vi "re_LuaVIEW Task State Machine.vi"   [LabVIEW 2012]
doc: "Implements a LuaVIEW task execution management: script compilation, execution, and default signal handling."
uses:
  typedefs/t_LuaVIEW Task States.ctl
  typedefs/t_LuaVIEW Task State Methods.ctl
  typedefs/t_LuaVIEW Task Signals.ctl
  typedefs/et_LuaVIEW CIN Actions.ctl
  typedefs/t_LuaVIEW Task Modes.ctl
  typedefs/t_LuaVIEW Task State Instantiator Methods.ctl
  typedefs/t_LuaVIEW Task List Methods.ctl
types:
  T1 = typedef "t_LuaVIEW Task States.ctl" = enum16{"handle signals", "test confirm", "test stop", "test swap", "test pause", "test resume", "sleep", "execute", "initialize", "list self", "set refs", "error", "stop"}
  T2 = typedef "t_LuaVIEW Task Signals.ctl" = enum32{"resume", "pause", "swap", "stop", "confirm"}
  T3 = typedef "t_LuaVIEW Task State Methods.ctl" = enum16{"cleanup", "set initial", "set mode", "set active mode", "set error", "get task info", "get script info", "set signal", "clear signal", "test handled", "test delegated", "test signal", "handle signal", "delegate signal", "allow signal", "disallow signal", "disallow all", "signals?", "delegated signals?", "protection++", "protection--", "protection=0", "message", "next message", "pop message", "message available?", "force stop", "set swap preps", "apply swap preps"}
  T4 = typedef "et_LuaVIEW CIN Actions.ctl" = enum16{"checksynopsis", "_open", "_registerpublic", "_registerexport", "__never_an_error_result_ns", "luaversion", "cinversion", "_totals", "_taskcount", "pathological", "_unregnextpublic", "registryusecount", "__per_state_actions", "regsetprivate", "regsetindex", "regsetmodule", "_revokeexports", "_usepublic", "prepare", "compile", "execute", "call", "unregstaterefs", "_close", "pullboolean", "pullnumber", "pullI8", "pullU8", "pullI16", "pullU16", "pullI32", "pullU32", "pullobject", "pullrefnum", "pullstring", "pullflat", "pushflat", "pushobject", "getattribute", "setattribute", "stacktostring", "_startyieldtest", "_endyieldtest", "_pollprintbuffer", "__never_an_error_result_ps", "_pollexport", "setclone", "forcecleanup", "gettop", "clearstack", "insert", "pushboolean", "pushnumber", "pushrefnum", "pushstring", "pushnil", "pushvalue", "gettaskref", "settaskref"}
  T5 = typedef "t_LuaVIEW Task Modes.ctl" = enum16{"initializing", "running", "executing", "paused", "error", "swapping"}
  T6 = typedef "t_LuaVIEW Task State Instantiator Methods.ctl" = enum16{"instantiate", "isset", "retrieve"}
  T7 = typedef "t_LuaVIEW Task List Methods.ctl" = enum16{"clear list", "add", "test", "remove", "get ref", "get task info", "get list", "get script info", "ongoing?", "resume", "pause", "stop", "confirm", "message"}
  T8 = typedef "t_LuaVIEW Task State Pane.ctl" = refnum<vi>
  T9 = typedef "t_LuaVIEW Reference.ctl" = refnum<k1>
  T10 = typedef "LuaVIEW Task Info.ctl" = cluster{"main script":string, "identifier":string, "class":string, "description":string, "mode":T5, "handler":string, "LuaVIEW reference":T9, "scripts":i32, "hide":bool, "active":bool, "error msg":string, "defer":bool, "launch":enum16{"asynchronous", "manual", "synchronous"}, "main path valid":bool, "start time":dbl, "swap time":dbl, "task VI":refnum<vi>, "prefsys":enum32{"invalid execution system", "user interface", "standard", "instrument i/o", "data acquisition", "other 1", "other 2", "same as caller"}, "priority":enum32{"invalid priority", "background priority", "normal priority", "above normal priority", "high priority", "time critical priority", "subroutine"}, "signal flags":u32, "allow mask":u32, "handle mask":u32, "disallow manual":bool}
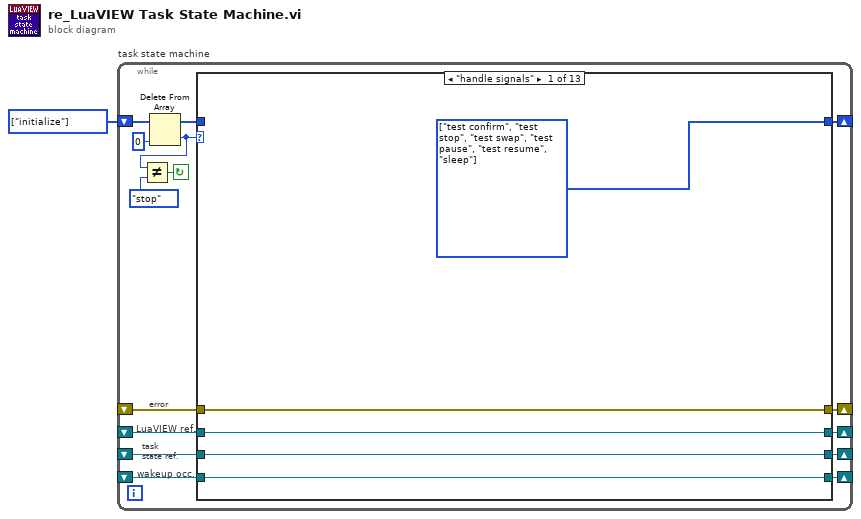
[diagram p0: block diagram]
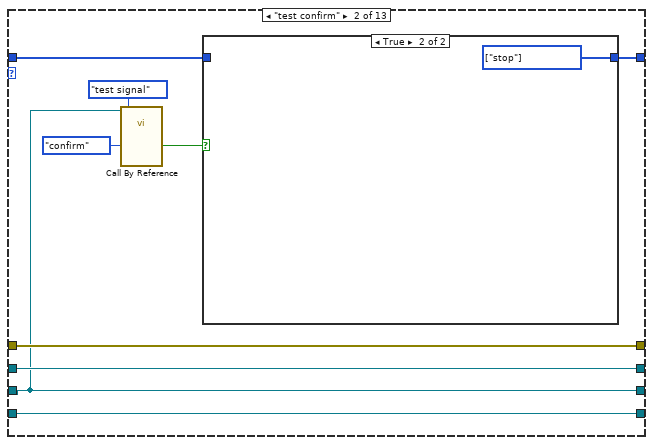
[diagram p2: hidden frame]
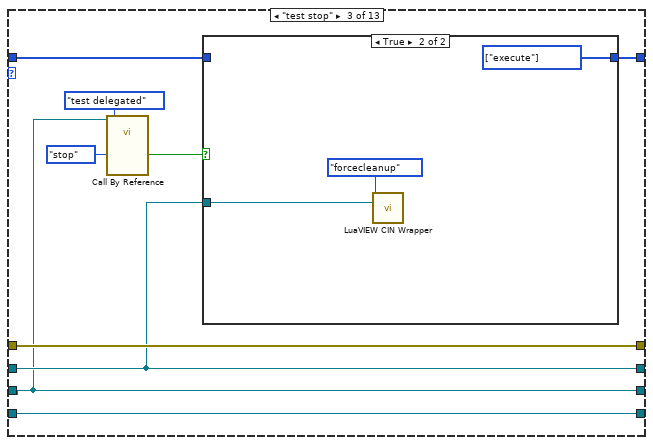
[diagram p4: hidden frame]
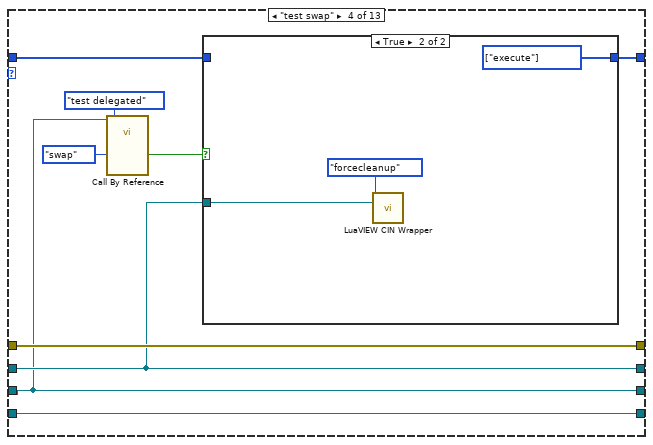
[diagram p6: hidden frame]
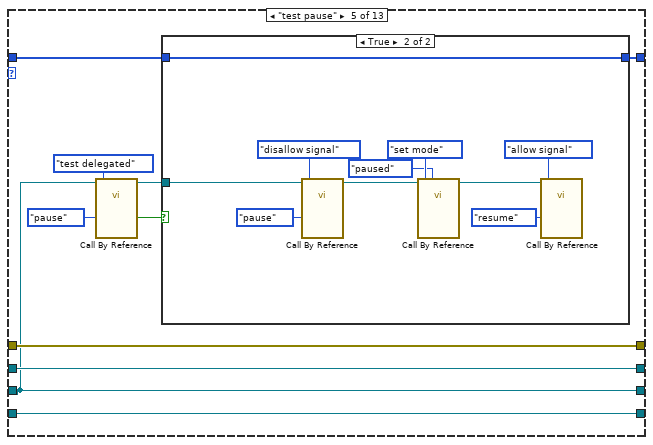
[diagram p8: hidden frame]
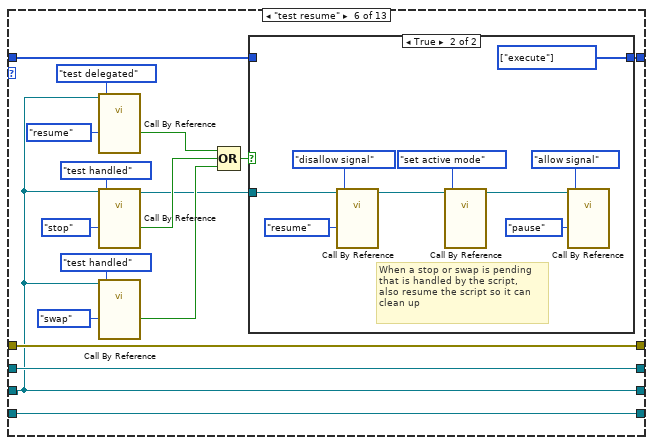
[diagram p10: hidden frame]
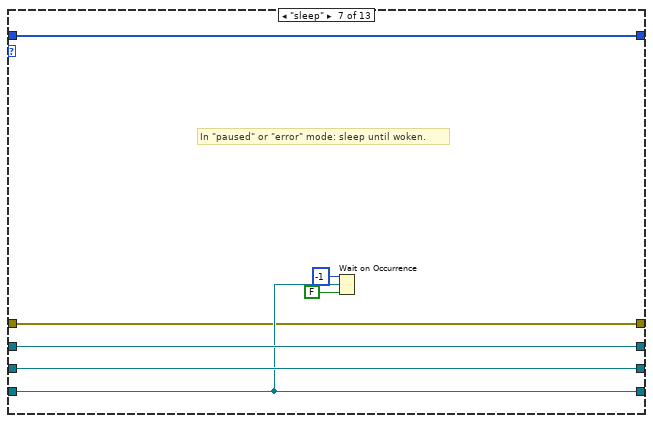
[diagram p12: hidden frame]
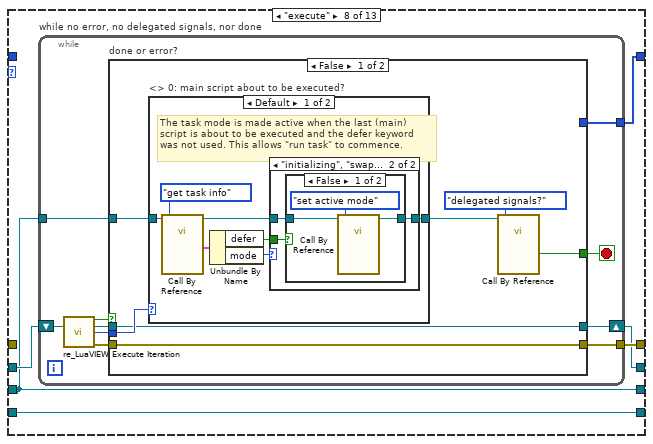
[diagram p13: hidden frame]
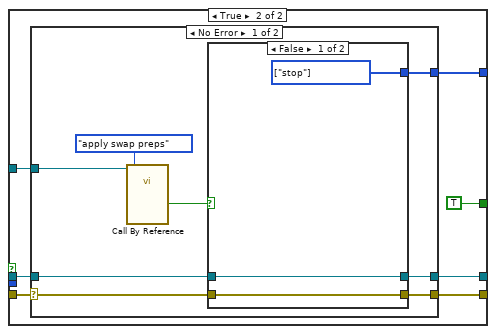
[diagram p17: hidden frame]
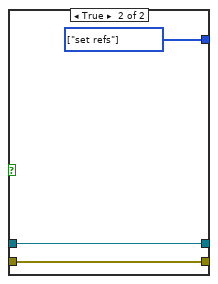
[diagram p18: hidden frame]
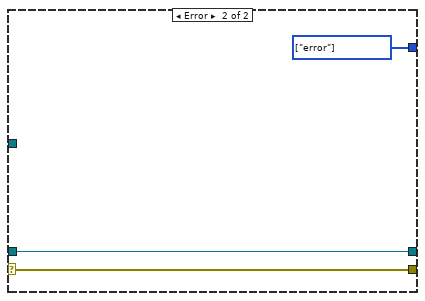
[diagram p19: hidden frame]
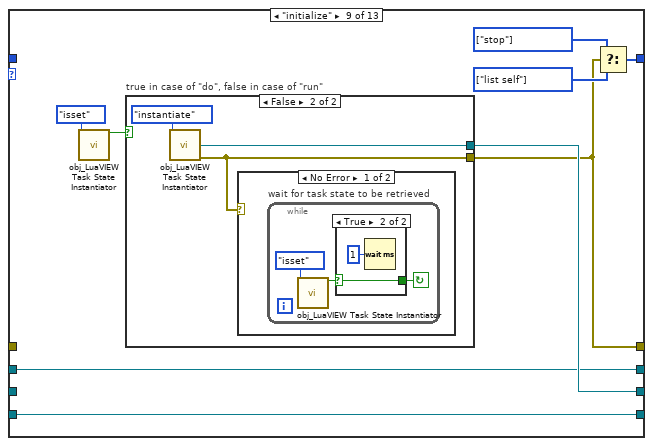
[diagram p20: hidden frame]
diagram:
  w1 = T1[] [enum."initialize"] items=["handle signals", "test confirm", "test stop", "test swap", "test pause", "test resume", "sleep", "execute", "initialize", "list self", "set refs", "error", "stop"] ("Array Constant")
  n1 = while "task state machine" {
    shift-left: w1 -> [w14]
    shift-right: [w7] -> _
    shift-right: [w11] -> _
    shift-left: _ -> [w8]
    shift-right: [w3] -> _
    shift-left: _ -> [w4]
    shift-right: [w10] -> _
    shift-left: _ -> [w9]
    shift-right: [w6] -> _
    shift-left: _ -> [w5]
    stop <- w16 continue-if-true
    # "error"
    # "LuaVIEW ref."
    # "task\nstate ref."
    # "wakeup occ."
    n2 = Delete From Array(array=w14, index=0) -> (deleted portion=w2:T1, array with subset deleted=w13:T1[])  [unwired: 1 in]
    n3 = Not Equal?(x=w2, y=t_LuaVIEW_Task_States."stop" ("states")) -> (x != y?=w16:bool)
    n4 = case "Case" shown="\"handle signals\"" w2 {
      tunnel: [w17 w27 w39 w52 w65 w93 w107 w115 w183 w199 w211 w218 w228] -> w7
      tunnel: w13 -> [_ w28 w40 w53 w66 w94 w107 _ _ _ _ _ w228]
      tunnel: [w20 w25 w36 w49 w60 w81 w112 w114 w180 w202 w208 w214 w222] -> w11
      tunnel: [w19 w29 w41 w54 w67 w95 w109 w117 w177 w198 w213 w220 w227] -> w10
      tunnel: w9 -> [w19 w29 w41 w54 w67 w95 w109 w117 w177 _ w213 w220 w227]
      tunnel: w8 -> [w20 w25 w36 w49 w60 w81 w112 w114 _ w202 w208 w214 w223]
      tunnel: [w21 w30 w37 w50 w68 w96 w113 w118 w178 w201 w206 w221 w226] -> w3
      tunnel: w4 -> [w21 w30 w37 w50 w68 w96 w113 w116 w178 w201 _ w221 w226]
      tunnel: [w18 w26 w38 w51 w64 w92 w108 w119 w179 w200 w212 w219 w225] -> w6
      tunnel: w5 -> [w18 w26 w38 w51 w64 w92 w108 _ _ w200 w212 w219 w225]
      frame "handle signals" {
        w17 = T1[] [enum."test confirm", enum."test stop", enum."test swap", enum."test pause", enum."test resume", enum."sleep"] items=["handle signals", "test confirm", "test stop", "test swap", "test pause", "test resume", "sleep", "execute", "initialize", "list self", "set refs", "error", "stop"] ("Array Constant")
      }
      frame "test confirm" {
        n5 = call-by-ref "?"(reference=w25, "method"=t_LuaVIEW_Task_State_Methods."test signal", "signal"=t_LuaVIEW_Task_Signals."confirm") -> ("set/available/pending"=w22:bool)  [unwired: 10 in, 6 out]
        n6 = case shown="True" w22 {
          tunnel: w28 -> [w31 _]
          tunnel: [w31 w32] -> w27
          frame False {
          }
          frame True {
            w32 = T1[] [enum."stop"] items=["handle signals", "test confirm", "test stop", "test swap", "test pause", "test resume", "sleep", "execute", "initialize", "list self", "set refs", "error", "stop"] ("Array Constant")
          }
        }
      }
      frame "test stop" {
        n7 = call-by-ref "?"(reference=w36, "method"=t_LuaVIEW_Task_State_Methods."test delegated", "signal"=t_LuaVIEW_Task_Signals."stop") -> ("set/available/pending"=w35:bool)  [unwired: 10 in, 6 out]
        n8 = case shown="True" w35 {
          tunnel: w40 -> [w42 _]
          tunnel: [w42 w45] -> w39
          tunnel: w37 -> [_ w43]
          frame False {
          }
          frame True {
            w45 = T1[] [enum."execute"] items=["handle signals", "test confirm", "test stop", "test swap", "test pause", "test resume", "sleep", "execute", "initialize", "list self", "set refs", "error", "stop"] ("Array Constant")
            n9 = call "LuaVIEW CIN Wrapper.vi"("action"=et_LuaVIEW_CIN_Actions."forcecleanup", "LuaVIEW reference in"=w43) -> ()  [unwired: 13 in, 1 out]
          }
        }
      }
      frame "test swap" {
        n10 = call-by-ref "?"(reference=w49, "method"=t_LuaVIEW_Task_State_Methods."test delegated", "signal"=t_LuaVIEW_Task_Signals."swap") -> ("set/available/pending"=w48:bool)  [unwired: 10 in, 6 out]
        n11 = case shown="True" w48 {
          tunnel: w53 -> [w55 _]
          tunnel: [w55 w58] -> w52
          tunnel: w50 -> [_ w56]
          frame False {
          }
          frame True {
            w58 = T1[] [enum."execute"] items=["handle signals", "test confirm", "test stop", "test swap", "test pause", "test resume", "sleep", "execute", "initialize", "list self", "set refs", "error", "stop"] ("Array Constant")
            n12 = call "LuaVIEW CIN Wrapper.vi"("action"=et_LuaVIEW_CIN_Actions."forcecleanup", "LuaVIEW reference in"=w56) -> ()  [unwired: 13 in, 1 out]
          }
        }
      }
      frame "test pause" {
        n13 = call-by-ref "?"(reference=w60, "method"=t_LuaVIEW_Task_State_Methods."test delegated", "signal"=t_LuaVIEW_Task_Signals."pause") -> (reference out=w59:T8, "set/available/pending"=w61:bool)  [unwired: 10 in, 5 out]
        n14 = case shown="True" w61 {
          tunnel: w66 -> [w69 w79]
          tunnel: [w69 w79] -> w65
          tunnel: w59 -> [_ w72]
          frame False {
          }
          frame True {
            n15 = call-by-ref "?"(reference=w72, "method"=t_LuaVIEW_Task_State_Methods."disallow signal", "signal"=t_LuaVIEW_Task_Signals."pause") -> (reference out=w71:T8)  [unwired: 10 in, 6 out]
            n16 = call-by-ref "?"(reference=w71, "method"=t_LuaVIEW_Task_State_Methods."set mode", "mode {set mode}"=t_LuaVIEW_Task_Modes."paused" ("mode")) -> (reference out=w70:T8)  [unwired: 10 in, 6 out]
            n17 = call-by-ref "?"(reference=w70, "method"=t_LuaVIEW_Task_State_Methods."allow signal", "signal"=t_LuaVIEW_Task_Signals."resume") -> ()  [unwired: 10 in, 7 out]
          }
        }
      }
      frame "test resume" {
        n18 = call-by-ref "?"(reference=w81, "method"=t_LuaVIEW_Task_State_Methods."test delegated", "signal"=t_LuaVIEW_Task_Signals."resume") -> ("set/available/pending"=w82:bool)  [unwired: 10 in, 6 out]
        n19 = call-by-ref "?"(reference=w81, "method"=t_LuaVIEW_Task_State_Methods."test handled", "signal"=t_LuaVIEW_Task_Signals."stop") -> (reference out=w80:T8, "set/available/pending"=w85:bool)  [unwired: 10 in, 5 out]
        n20 = call-by-ref "?"(reference=w81, "method"=t_LuaVIEW_Task_State_Methods."test handled", "signal"=t_LuaVIEW_Task_Signals."swap") -> ("set/available/pending"=w88:bool)  [unwired: 10 in, 6 out]
        n21 = Compound Arithmetic op=OR(w82, w85, w88) -> (w91:bool)
        n22 = case shown="True" w91 {
          tunnel: w94 -> [w97 _]
          tunnel: [w97 w106] -> w93
          tunnel: w80 -> [_ w98]
          frame False {
          }
          frame True {
            w106 = T1[] [enum."execute"] items=["handle signals", "test confirm", "test stop", "test swap", "test pause", "test resume", "sleep", "execute", "initialize", "list self", "set refs", "error", "stop"] ("Array Constant")
            # "When a stop or swap is pending\nthat is handled by the script,\nalso resume the script so it can\nclean up"
            n23 = call-by-ref "?"(reference=w98, "method"=t_LuaVIEW_Task_State_Methods."disallow signal", "signal"=t_LuaVIEW_Task_Signals."resume") -> (reference out=w100:T8)  [unwired: 10 in, 6 out]
            n24 = call-by-ref "?"(reference=w100, "method"=t_LuaVIEW_Task_State_Methods."set active mode") -> (reference out=w99:T8)  [unwired: 11 in, 6 out]
            n25 = call-by-ref "?"(reference=w99, "method"=t_LuaVIEW_Task_State_Methods."allow signal", "signal"=t_LuaVIEW_Task_Signals."pause") -> ()  [unwired: 10 in, 7 out]
          }
        }
      }
      frame "sleep" {
        # "In \"paused\" or \"error\" mode: sleep until woken."
        n26 = Wait on Occurrence(1:FALSE ("ignore previous (T)"), 2:w109, 3:-1 ("ms timeout (-1)")) -> ()  [unwired: 1 out]
      }
      frame "execute" {
        n27 = while "while no error, no delegated signals, nor done" {
          shift-right: [w129] -> w118
          shift-left: w116 -> [w123]
          tunnel: [w128] -> w119
          tunnel: [w121] -> w115
          tunnel: w114 -> [w120]
          stop <- w127 stop-if-true
          n28 = call "re_LuaVIEW Execute Iteration.vi"("LuaVIEW reference in"=w123) -> ("last?"=w122:bool, "LuaVIEW reference out"=w125:T9, "function index"=w126:i32, "final error"=w124:errorcluster)  [unwired: 11 in]
          n29 = case "done or error?" shown="False" w122 {
            tunnel: [w135 w155] -> w129
            tunnel: [w134 w158] -> w128
            tunnel: [w133 TRUE] -> w127
            tunnel: w126 -> [w136 _]
            tunnel: w125 -> [w135 w156]
            tunnel: w124 -> [w134 w159]
            tunnel: [_ w157] -> w121
            tunnel: w120 -> [w132 w153]
            frame False {
              n30 = case "<> 0: main script about to be executed?" shown="Default" w136 {
                tunnel: w132 -> [w139 w152]
                tunnel: [w137 w152] -> w131
                frame Default {
                  # "The task mode is made active when the last (main)\nscript is about to be executed and the defer keyword\nwas not used. This allows \"run task\" to commence."
                  n31 = call-by-ref "?"(reference=w139, "method"=t_LuaVIEW_Task_State_Methods."get task info") -> (reference out=w138:T8, "task info {get task info}"=w141:T10)  [unwired: 11 in, 5 out]
                  n32 = Unbundle By Name(w141) -> ("defer"=w142:bool, "mode"=w143:T5)
                  n33 = case shown="\"initializing\", \"swapping\"" w143 {
                    tunnel: w142 -> [_ w147]
                    tunnel: w138 -> [w144 w146]
                    tunnel: [w144 w145] -> w137
                    frame Default {
                    }
                    frame "initializing", "swapping" {
                      n34 = case shown="False" w147 {
                        tunnel: w146 -> [w149 w151]
                        tunnel: [w148 w151] -> w145
                        frame False {
                          n35 = call-by-ref "?"(reference=w149, "method"=t_LuaVIEW_Task_State_Methods."set active mode") -> (reference out=w148:T8)  [unwired: 11 in, 6 out]
                        }
                        frame True {
                        }
                      }
                    }
                  }
                }
                frame 0 {
                }
              }
              n36 = call-by-ref "?"(reference=w131, "method"=t_LuaVIEW_Task_State_Methods."delegated signals?") -> ("set/available/pending"=w133:bool)  [unwired: 11 in, 6 out]
            }
            frame True {
              n37 = case shown="No Error" w159 {
                selector: w159 -> [w164 w176]
                tunnel: [w163 w176] -> w158
                tunnel: [w167 w175] -> w157
                tunnel: w156 -> [w166 w174]
                tunnel: [w165 w174] -> w155
                tunnel: w153 -> [w161 _]
                frame No Error {
                  n38 = call-by-ref "?"(reference=w161, "method"=t_LuaVIEW_Task_State_Methods."apply swap preps") -> ("set/available/pending"=w160:bool)  [unwired: 11 in, 6 out]
                  n39 = case shown="False" w160 {
                    tunnel: [w170 w171] -> w167
                    tunnel: w166 -> [w169 w173]
                    tunnel: [w169 w173] -> w165
                    tunnel: w164 -> [w168 w172]
                    tunnel: [w168 w172] -> w163
                    frame False {
                      w170 = T1[] [enum."stop"] items=["handle signals", "test confirm", "test stop", "test swap", "test pause", "test resume", "sleep", "execute", "initialize", "list self", "set refs", "error", "stop"] ("Array Constant")
                    }
                    frame True {
                      w171 = T1[] [enum."set refs"] items=["handle signals", "test confirm", "test stop", "test swap", "test pause", "test resume", "sleep", "execute", "initialize", "list self", "set refs", "error", "stop"] ("Array Constant")
                    }
                  }
                }
                frame Error {
                  w175 = T1[] [enum."error"] items=["handle signals", "test confirm", "test stop", "test swap", "test pause", "test resume", "sleep", "execute", "initialize", "list self", "set refs", "error", "stop"] ("Array Constant")
                }
              }
            }
          }
        }
      }
      frame "initialize" {
        w184 = T1[] [enum."list self"] items=["handle signals", "test confirm", "test stop", "test swap", "test pause", "test resume", "sleep", "execute", "initialize", "list self", "set refs", "error", "stop"] ("Array Constant")
        w185 = T1[] [enum."stop"] items=["handle signals", "test confirm", "test stop", "test swap", "test pause", "test resume", "sleep", "execute", "initialize", "list self", "set refs", "error", "stop"] ("Array Constant")
        n40 = call "obj_LuaVIEW Task State Instantiator.vi"("method"=t_LuaVIEW_Task_State_Instantiator_Methods."isset") -> ("set for retrieval?"=w181:bool)  [unwired: 12 in, 2 out]
        n41 = case "true in case of \"do\", false in case of \"run\"" shown="False" w181 {
          tunnel: [w187 w189] -> w179
          tunnel: [w186 w190] -> w180
          frame True {
            n42 = call "obj_LuaVIEW Task State Instantiator.vi"("method"=t_LuaVIEW_Task_State_Instantiator_Methods."retrieve") -> ("state object ref"=w186:T8, "instantiation error"=w187:errorcluster)  [unwired: 12 in, 1 out]
          }
          frame False {
            n43 = call "obj_LuaVIEW Task State Instantiator.vi"("method"=t_LuaVIEW_Task_State_Instantiator_Methods."instantiate") -> ("state object ref"=w190:T8, "instantiation error"=w189:errorcluster)  [unwired: 12 in, 1 out]
            n44 = case shown="No Error" w189 {
              frame No Error {
                n45 = while "wait for task state to be retrieved" {
                  stop <- w192 continue-if-true
                  n46 = call "obj_LuaVIEW Task State Instantiator.vi"("method"=t_LuaVIEW_Task_State_Instantiator_Methods."isset") -> ("set for retrieval?"=w193:bool)  [unwired: 12 in, 2 out]
                  n47 = case shown="True" w193 {
                    selector: w193 -> [w195 w196]
                    tunnel: [w195 w196] -> w192
                    frame False {
                    }
                    frame True {
                      n48 = Wait (ms)(milliseconds to wait=u32 1) -> ()  [unwired: 1 out]
                    }
                  }
                }
              }
              frame Error {
              }
            }
          }
        }
        n49 = Select(t=w185, s=w179, f=w184) -> (s? t:f=w183:T1[])
      }
      frame "list self" {
        w199 = T1[] [enum."set refs"] items=["handle signals", "test confirm", "test stop", "test swap", "test pause", "test resume", "sleep", "execute", "initialize", "list self", "set refs", "error", "stop"] ("Array Constant")
        n50 = call "obj_LuaVIEW Task List.vi"("method"=t_LuaVIEW_Task_List_Methods."add", "state object ref in"=w202) -> ("wakeup occurrence"=w198:refnum<k4>)  [unwired: 8 in, 5 out]
      }
      frame "set refs" {
        w211 = T1[] [enum."execute"] items=["handle signals", "test confirm", "test stop", "test swap", "test pause", "test resume", "sleep", "execute", "initialize", "list self", "set refs", "error", "stop"] ("Array Constant")
        n51 = call-by-ref "?"(reference=w208, "method"=t_LuaVIEW_Task_State_Methods."get task info") -> ("task info {get task info}"=w209:T10)  [unwired: 11 in, 6 out]
        n52 = Unbundle By Name(w209) -> ("LuaVIEW reference"=w205:T9)
        n53 = call "LuaVIEW Cast VI Ref to Gen Ref.vi"("refnum in"=w208) -> ("refnum out"=w207:refnum<vi>)  [unwired: 14 in]
        n54 = call "LuaVIEW CIN Wrapper.vi"("action"=et_LuaVIEW_CIN_Actions."settaskref", "refnum in"=w207, "LuaVIEW reference in"=w205) -> ("LuaVIEW reference out"=w206:T9)  [unwired: 12 in]
      }
      frame "error" {
        w216 = T1[] [enum."sleep"] items=["handle signals", "test confirm", "test stop", "test swap", "test pause", "test resume", "sleep", "execute", "initialize", "list self", "set refs", "error", "stop"] ("Array Constant")
        w217 = T1[] [enum."stop"] items=["handle signals", "test confirm", "test stop", "test swap", "test pause", "test resume", "sleep", "execute", "initialize", "list self", "set refs", "error", "stop"] ("Array Constant")
        n55 = call "LuaVIEW Handle Task Error.vi"("state object ref"=w214, "error"=w219) -> ("cleanup?"=w215:bool)  [unwired: 13 in]
        n56 = Select(t=w217, s=w215, f=w216) -> (s? t:f=w218:T1[])
      }
      frame "stop" {
        n57 = Not A Number/Path/Refnum?(number/path/refnum=w223) -> (NaN/Path/Refnum?=w224:bool)
        n58 = case shown="False" w224 {
          tunnel: w223 -> [w234 w240]
          tunnel: [_ w240] -> w222
          frame False {
            n59 = call-by-ref "?"(reference=w234, "method"=t_LuaVIEW_Task_State_Methods."get task info") -> (reference out=w233:T8, "task info {get task info}"=w236:T10)  [unwired: 11 in, 5 out]
            n60 = Unbundle By Name(w236) -> ("launch"=w229:enum16{"asynchronous", "manual", "synchronous"})
            n61 = stacked-sequence {
              tunnel: w233 -> [w237]
              tunnel: [w237] -> w231
              frame #0 {
                n62 = call "obj_LuaVIEW Task List.vi"("method"=t_LuaVIEW_Task_List_Methods."remove", "state object ref in"=w237) -> ()  [unwired: 8 in, 6 out]
              }
            }
            n63 = call-by-ref "?"(reference=w231, "method"=t_LuaVIEW_Task_State_Methods."cleanup") -> (reference out=w230:T8)  [unwired: 11 in, 6 out]
            n64 = case shown="\"synchronous\"" w229 {
              tunnel: w230 -> [_ w239]
              frame "synchronous" {
                # "launching context\nhas instantiated\nthe state and is\nresponsible for\nclosing its ref."
              }
              frame Default {
                n65 = Close Reference(reference=w239) -> ()  [unwired: 1 in, 1 out]
              }
            }
          }
          frame True {
          }
        }
      }
    }
  }
